vi "Configure Pulse.vi"(0 "VISA resource name":refnum<visa-resource-name>, 5 "Enable Continuous Pulses (F: Disable)":bool, 7 "Pulse Count (1)":dbl=1.0 format="%#.4g", 9 "Period (0.0333 s)":dbl=0.03333 format="%#.4g", 11 "error in (no error)":errorcluster, 12 "Pulse Characteristic (0: Duty Cycle)":u16(ring) items=["Duty Cycle", "Pulse Width"], 13 "Pulse Characteristic Value (50)":dbl=50.0 format="%#.4g") -> (4 "VISA resource name out":refnum<visa-resource-name>, 15 "error out":errorcluster)   [LabVIEW 2019, in "Agilent 681x Series.lvlib"]
doc: "Specifies the pulse characteristics and uses a user-defined pulse characteristic (period or width) to allow the instrument to calculate the other automatically."
uses:
  <instrlib>/Agilent 681x Series/Agilent 681x Series.lvlib
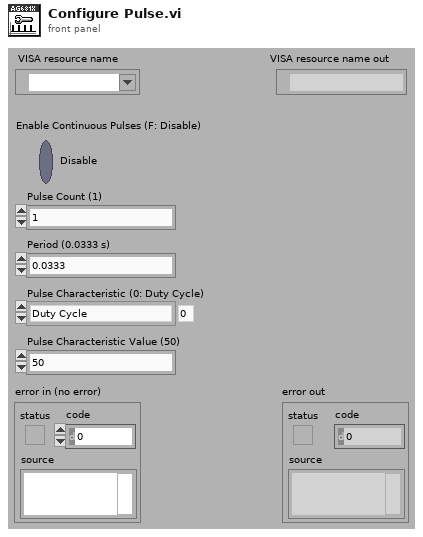
[diagram p1: front panel]
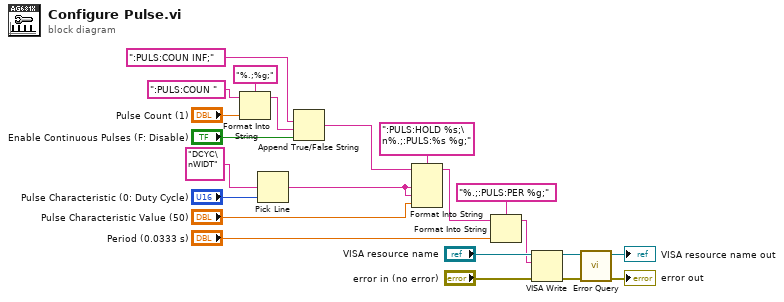
[diagram p0: block diagram]
diagram:
  n1 = Format Into String(format string="%.;%g;", initial string=":PULS:COUN ", "Pulse Count (1)") -> (resulting string=w14:string)  [unwired: 1 in, 1 out]
  n2 = Pick Line(multi-line string="DCYC\nWIDT" ("true string"), line index="Pulse Characteristic (0: Duty Cycle)") -> (output string=w1:string)  [unwired: 1 in]
  n3 = Append True/False String(1:"Enable Continuous Pulses (F: Disable)", 2:w14, 3:":PULS:COUN INF;" ("false string")) -> (0:w6:string)  [unwired: 1 in]
  n4 = Format Into String(format string=":PULS:HOLD %s;\n%.;:PULS:%s %g;", initial string=w6, w1, w1, "Pulse Characteristic Value (50)") -> (resulting string=w4:string)  [unwired: 1 in, 1 out]
  n5 = Format Into String(format string="%.;:PULS:PER %g;", initial string=w4, "Period (0.0333 s)") -> (resulting string=w8:string)  [unwired: 1 in, 1 out]
  n6 = VISA Write(VISA resource name="VISA resource name", write buffer=w8, error in (no error)="error in (no error)") -> (VISA resource name out=w20:refnum<visa-resource-name>, error out=w19:errorcluster)  [unwired: 1 out]
  n7 = call <instrlib>:"Error Query.vi"("error in (no error)"=w19, "VISA resource name"=w20) -> ("error out"=→"error out":errorcluster, "VISA resource name out"=→"VISA resource name out":refnum<visa-resource-name>)  [unwired: 6 in, 2 out]
